vi "user intialization.vi"(8 "error in":errorcluster, 10 "configuration in":refnum<class "control module configuration.lvclass">, 11 "fixed channel runtime in":refnum<class "control module runtime.lvclass">) -> (0 "error out":errorcluster, 3 "fixed channel runtime out":refnum<class "control module runtime.lvclass">)   [LabVIEW 2013, in "control module runtime.lvclass"]
uses:
  control module runtime.lvclass
  configuration/control module configuration.lvclass
  configuration/control module configuration.lvclass/control module configuration.ctl
  control module runtime.lvclass/control module runtime.ctl
  configuration/Read error classifications.vi
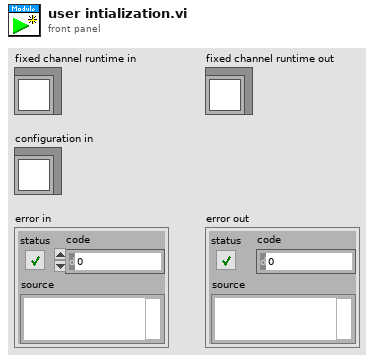
[diagram p1: front panel]
types:
  T1 = typedef "control module configuration.lvclass/error classification.ctl" = cluster{"code":i32, "error classification":T2}
  T2 = typedef "TBM module execution interface.lvclass/error classification.ctl" = enum16{"unknown", "none", "trivial", "recoverable", "critical"}
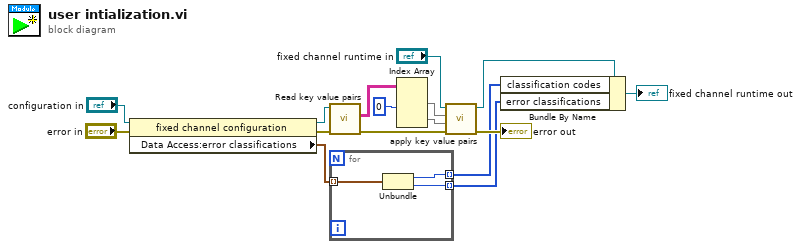
[diagram p0: block diagram]
diagram:
  n1 = property class="fixed channel configuration"(reference="configuration in", error in="error in") -> (reference out=w4:refnum<class "control module configuration.lvclass">, error out=w6:errorcluster, "Data Access:error classifications"=w3:T1[])
  n2 = call "Read key value pairs.vi"("error in"=w6, "fixed channel configuration in"=w4) -> ("error out"=w11:errorcluster, "key value pairs"=w16:string[][])  [unwired: 7 in, 1 out]
  n3 = for {
    tunnel: w3 -> [w19] mode=indexing
    tunnel: [w18] -> w2 mode=indexing
    tunnel: [w17] -> w1 mode=indexing
    n4 = Unbundle(w19) -> ("code"=w18:i32, "error classification"=w17:T2)
  }
  n5 = Index Array(array=w16, index (col) #1=0 ("disabled index (col)")) -> (element #1=w9:string[], element #2=w8:string[])  [unwired: 3 in]
  n6 = call-dynamic "apply key value pairs.vi"("error in"=w11, "values"=w8, "keys"=w9, "fixed channel runtime in"="fixed channel runtime in") -> ("error out"=→"error out":errorcluster, "fixed channel runtime out"=w12:refnum<class "control module runtime.lvclass">)  [unwired: 6 in]
  n7 = Bundle By Name(cluster=w12, "classification codes"=w2, "error classifications"=w1) -> (→"fixed channel runtime out":refnum<class "control module runtime.lvclass">)
